vi "Set Sense Connection.vi"(8 "error in (no error)":errorcluster, 10 "Sense Connection (T: Internal)":bool=TRUE, 11 "VISA resource name":refnum<visa-resource-name>) -> (0 "error out":errorcluster, 3 "VISA resource name out":refnum<visa-resource-name>)   [LabVIEW 2014, in "Fluke 5XXX Series Multicalibrators.lvlib"]
doc: "This VI selects internal or external sensing. (The same as pressing EX SNS in local operation.)\n\nNote:\n\nThis VI is available only for instrument models 5700A, 5720A and 57LFC."
uses:
  Fluke 5XXX Series Multicalibrators.lvlib
panel:
  # "Internal"
  # "External"
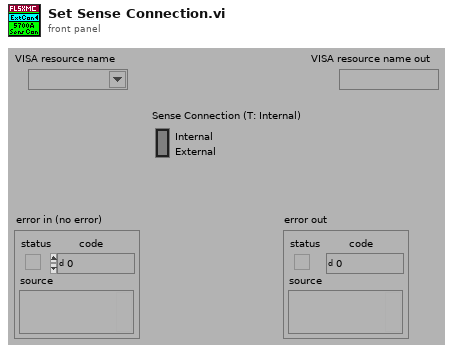
[diagram p1: front panel]
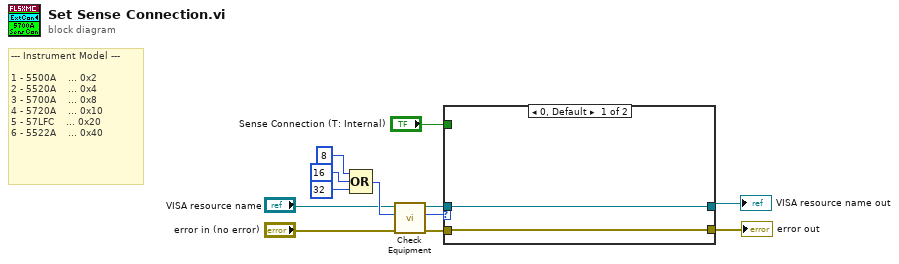
[diagram p0: block diagram]
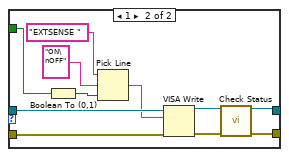
[diagram p2: hidden frame]
diagram:
  # "--- Instrument Model ---\n\n1 - 5500A    ... 0x2\n2 - 5520A    ... 0x4\n3 - 5700A    ... 0x8\n4 - 5720A    ... 0x10\n5 - 57LFC    ... 0x20\n6 - 5522A    ... 0x40"
  n1 = Compound Arithmetic op=OR(8 ("Numeric"), 16 ("Numeric"), 32 ("Numeric")) -> (w7:i32)
  n2 = call "Check Equipment.vi"("error in (no error)"="error in (no error)", "Bit Mask"=w7, "VISA resource name"="VISA resource name") -> ("error out"=w12:errorcluster, "Present?"=w11:u32, "VISA resource name out"=w10:refnum<visa-resource-name>)  [unwired: 6 in]
  n3 = case shown="0, Default" w11 {
    tunnel: "Sense Connection (T: Internal)" -> [_ w22]
    tunnel: [w13 w17] -> w2
    tunnel: w12 -> [w14 w21]
    tunnel: w10 -> [w13 w20]
    tunnel: [w14 w18] -> w3
    frame 0, Default {
    }
    frame 1 {
      n4 = Boolean To (0,1)(Boolean=w22) -> (0, 1=w23:i16)
      n5 = Pick Line(string ("")="EXTSENSE " ("Reset Command"), multi-line string="ON\nOFF", line index=w23) -> (output string=w19:string)
      n6 = VISA Write(VISA resource name=w20, write buffer=w19, error in (no error)=w21) -> (VISA resource name out=w16:refnum<visa-resource-name>, error out=w15:errorcluster)  [unwired: 1 out]
      n7 = call "Check Status.vi"("VISA resource name"=w16, "error in (no error)"=w15) -> ("VISA resource name out"=w17:refnum<visa-resource-name>, "error out"=w18:errorcluster)  [unwired: 12 in]
    }
  }
  "VISA resource name out" <- w2
  "error out" <- w3
